vi "采配水参数设置.vi"() -> ()   [LabVIEW 2016, in "环境动力单元.lvlib"]
uses:
  <vilib>/Utility/config.llb/NI_LVConfig.lvlib
panel:
  in  "布尔":bool
  out "沉淀时间":dbl=1800.0
  out "进样超时时间":dbl=300.0
  out "润洗时间":dbl=60.0
  out "排空时间":dbl=60.0
  # "参数设置"
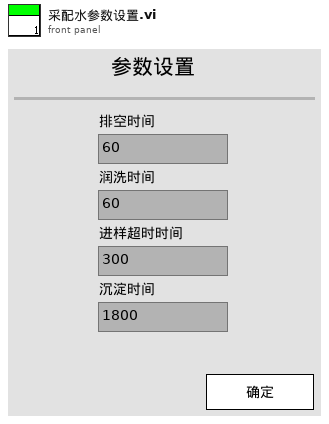
[diagram p1: front panel]
types:
  T1 = cluster{"排空时间":dbl, "润洗时间":dbl, "进样超时时间":dbl, "沉淀时间":dbl}
  T2 = typedef "NI_LVConfig.lvlib/Config Data RefNum.ctl" = refnum<k1>
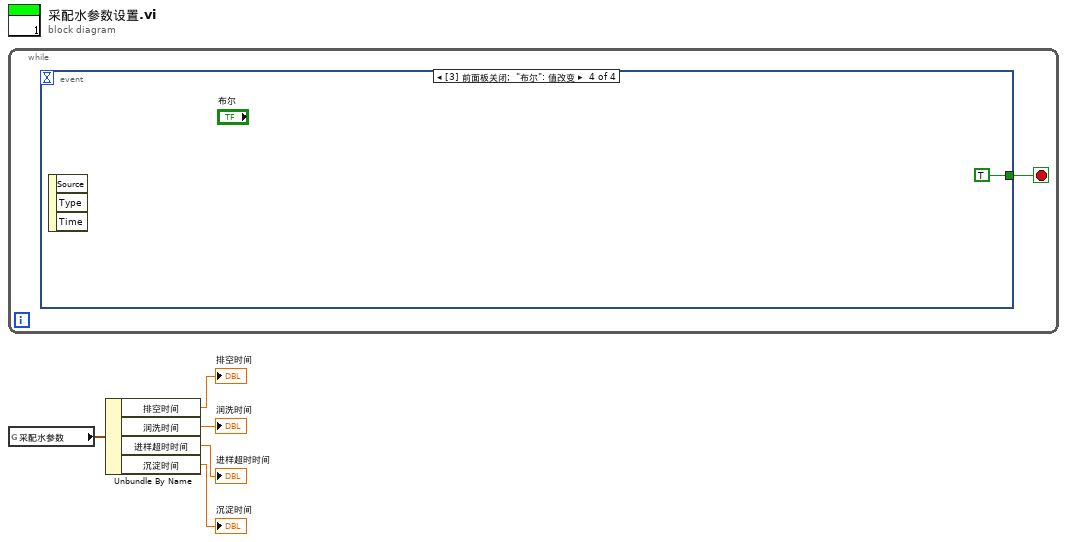
[diagram p0: block diagram]
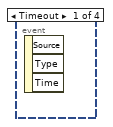
[diagram p2: hidden frame]
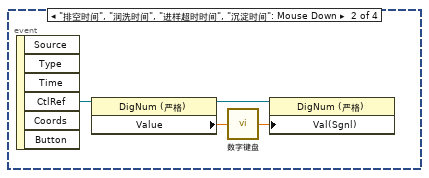
[diagram p3: hidden frame]
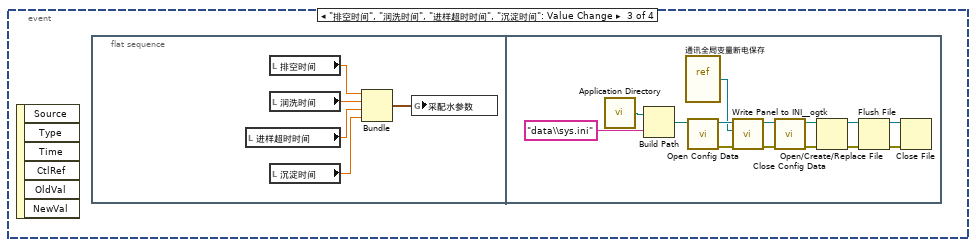
[diagram p4: hidden frame]
diagram:
  n1 = while {
    stop <- w6 stop-if-true
    n2 = event shown="[3] 前面板关闭;  \"布尔\": 值改变" {
      selector: _ -> [_ _ _ _]
      dyn-events: _ -> [_ _ _ _]
      timeout: _ -> [_ _ _ _]
      tunnel: [_ _ _ TRUE] -> w6
      event Timeout {
        n3 = event-data() -> ()  [unwired: 1 in, 3 out]
      }
      event "排空时间", "润洗时间", "进样超时时间", "沉淀时间": Mouse Down {
        n4 = event-data() -> ("CtlRef"=w10:refnum<vi>)  [unwired: 1 in, 5 out]
        n5 = property class="DigNum (严格)"(reference=w10) -> (reference out=w7:refnum<vi>, "Value"=w9:dbl)  [unwired: 1 in, 1 out]
        n6 = call "数字键盘.vi"("OldNumber"=w9) -> ("NewNumber"=w8:dbl)
        n7 = property class="DigNum (严格)"(reference=w7, "Val(Sgnl)"=w8) -> ()  [unwired: 1 in, 2 out]
      }
      event "排空时间", "润洗时间", "进样超时时间", "沉淀时间": Value Change {
        n8 = event-data() -> ()  [unwired: 1 in, 6 out]
        n9 = flat-sequence {
          frame #0 {
            n10 = local read "进样超时时间"() -> (w13:dbl)
            n11 = local read "排空时间"() -> (w15:dbl)
            n12 = local read "润洗时间"() -> (w14:dbl)
            n13 = local read "沉淀时间"() -> (w12:dbl)
            n14 = Bundle("排空时间"=w15, "润洗时间"=w14, "进样超时时间"=w13, "沉淀时间"=w12) -> (w11:T1)  [unwired: 1 in]
            n15 = global write "通讯全局变量断电保存.vi" "采配水参数"(w11) -> ()
          }
          frame #1 {
            n16 = call <vilib>:"Application Directory.vi"() -> ("Application Directory"=w29:path)
            n17 = Build Path(base path=w29, name or relative path="data\\sys.ini" ("名称或相对路径")) -> (appended path=w27:path)
            n18 = vi-ref "通讯全局变量断电保存.vi"() -> (w25:refnum<vi>)
            n19 = call <vilib>:"Open Config Data.vi"("configuration file path"=w27) -> ("error out"=w23:errorcluster, "refnum"=w26:T2)  [unwired: 8 in, 1 out]
            n20 = call <userlib>:"Write Panel to INI__ogtk.vi"("error in (no error)"=w23, "VI ref"=w25, "refnum"=w26) -> ("error out"=w22:errorcluster, "refnum out"=w24:T2)  [unwired: 7 in]
            n21 = call <vilib>:"Close Config Data.vi"("error in (no error)"=w22, "refnum"=w24) -> ("error out"=w17:errorcluster, "file path"=w16:path)  [unwired: 8 in]
            n22 = Open/Create/Replace File(file path (use dialog)=w16, error in=w17) -> (refnum out=w20:refnum<file>, error out=w21:errorcluster)  [unwired: 4 in, 1 out]
            n23 = Flush File(refnum=w20, error in=w21) -> (refnum out=w19:refnum<file>, error out=w18:errorcluster)
            n24 = Close File(refnum=w19, error in=w18) -> ()  [unwired: 2 out]
          }
        }
      }
      event Panel Close; "布尔": Value Change {
        n25 = event-data() -> ()  [unwired: 1 in, 3 out]
      }
    }
  }
  n26 = global read "通讯全局变量断电保存.vi" "采配水参数"() -> (w5:T1)
  n27 = Unbundle By Name(w5) -> ("排空时间"=→"排空时间":dbl, "润洗时间"=→"润洗时间":dbl, "进样超时时间"=→"进样超时时间":dbl, "沉淀时间"=→"沉淀时间":dbl)
